vi "MagBoard_Processor.vi"() -> ()   [LabVIEW 2018]
uses:
  <vilib>/Math Plots/3D Math Plots/3D Surface/3D Surface XCtrl/3D Surface.xctl
  <vilib>/Math Plots/3D Math Plots/3D Surface/3D Surface Datatype/3D Surface Datatype.lvclass
  subVIs/calibration/FGVs/FGV States.ctl
  <vilib>/Utility/file.llb/Write Delimited Spreadsheet (DBL).vi
  <vilib>/Math Plots/3D Math Plots/3D Surface/3D Surface Datatype/Public/Plot Helper (Matrix).vi
panel:
  in  "Calibration File":string="6x0-5mm"
  in  "Save Data":bool=TRUE
  in  "Export File (CSV)":path=path "C:/Users/menprc/Documents/GitHub/MagLib/MagBoard_n64_UI/MagBoard_n64_UI_LabVIEW_Client/example_data/M064_008.csv"
  in  "dT":u32=10
  in  "Tare":bool
  out "Node XYZ List":dbl[][](array[numeric])=[[-42.056, -3144.437, -23232.0], [-518.941, -325.183, -18275.84], [1216.62, -292.139, -19514.88], [1218.122, -1916.552, -21992.96], [2617.986, -1190.335, -20444.16], [-208.027, -4484.2210000000005, -19514.88], [258.344, 873.413, -19205.12], [-4699.758, -4066.665, -21373.44], [-165.971, -412.299, -24161.28], [-1390.852, 654.872, -16107.52], [519.692, -438.584, -21063.68], [-4446.671, -1839.95, -15178.24], [-2791.467, -3060.325, -17966.079999999998], [-4864.227, -3147.441, -15178.24], [-5380.164, -1542.554, -18585.6], [-829.104, -4714.778, -20753.92], [-2151.615, 1918.805, -22302.72], [-715.703, -1658.208, -21373.44], [-5288.542, -211.782, -15797.76], [-5200.675, -1924.062, -17346.559999999998], [-6355.713, -24.783, -16727.04], [-5830.764, -1267.688, -17346.559999999998], [-6334.685, -2507.589, -17036.8], [-5066.997, 553.487, -19514.88], [3860.891, 798.313, -17346.559999999998], [2385.927, -2710.359, -17346.559999999998], [573.764, -142.69, -27878.399999999998], [2370.907, 849.381, -16107.52], [1947.343, -7.51, -17656.32], [-2110.31, -343.958, -15797.76], [1126.5, -1583.859, -20753.92], [-2659.291, -2612.729, -20753.92], [-198.264, -502.419, -22302.72], [-2278.534, 1049.898, -17346.559999999998], [3332.938, 1936.078, -17346.559999999998], [-3211.276, 720.209, -17036.8], [-1516.269, 1041.637, -18275.84], [-1339.033, 228.304, -18585.6], [-4662.959, -1410.378, -18585.6], [-4996.403, -24.783, -16417.28], [1106.974, 4200.343, -20444.16], [1601.132, 2834.274, -19824.64], [-1445.675, 4241.648, -21373.44], [-953.019, 1932.323, -16727.04], [-1794.89, 2164.382, -21063.68], [-1591.369, 1783.625, -18585.6], [-2428.734, 724.715, -16727.04], [-4816.914, -1074.681, -23541.76], [1203.102, -101.385, -23541.76], [-2397.192, 482.142, -20753.92], [-4661.457, 7558.815, -16417.28], [-6119.148, 744.241, -16727.04], [-5919.382, -162.216, -19824.64], [-3782.036, -621.077, -15797.76], [-4665.212, -1492.237, -20134.399999999998], [-3349.46, -114.903, -17346.559999999998], [-3365.982, 4614.895, -22302.72], [-3110.642, 2824.511, -19205.12], [-2347.626, 20.277, -19514.88], [-533.21, -4829.681, -27258.879999999997], [-793.056, 5227.711, -24780.8], [-5263.759, 5650.524, -21992.96], [-3424.56, 3160.208, -18895.36], [-5248.739, 1337.531, -24161.28]]
  out "Time":u32=4294745741
  in  "stop":bool
  in  "Data File":path=path "C:/Users/menprc/Documents/GitHub/MagLib/MagBoard_n64_UI/MagBoard_n64_UI_LabVIEW_Client/example_data/M064_008_up.dat"
  out "Instantaneous Data":refnum<class "3D Plot Datatype.lvclass">[](xcontrol)
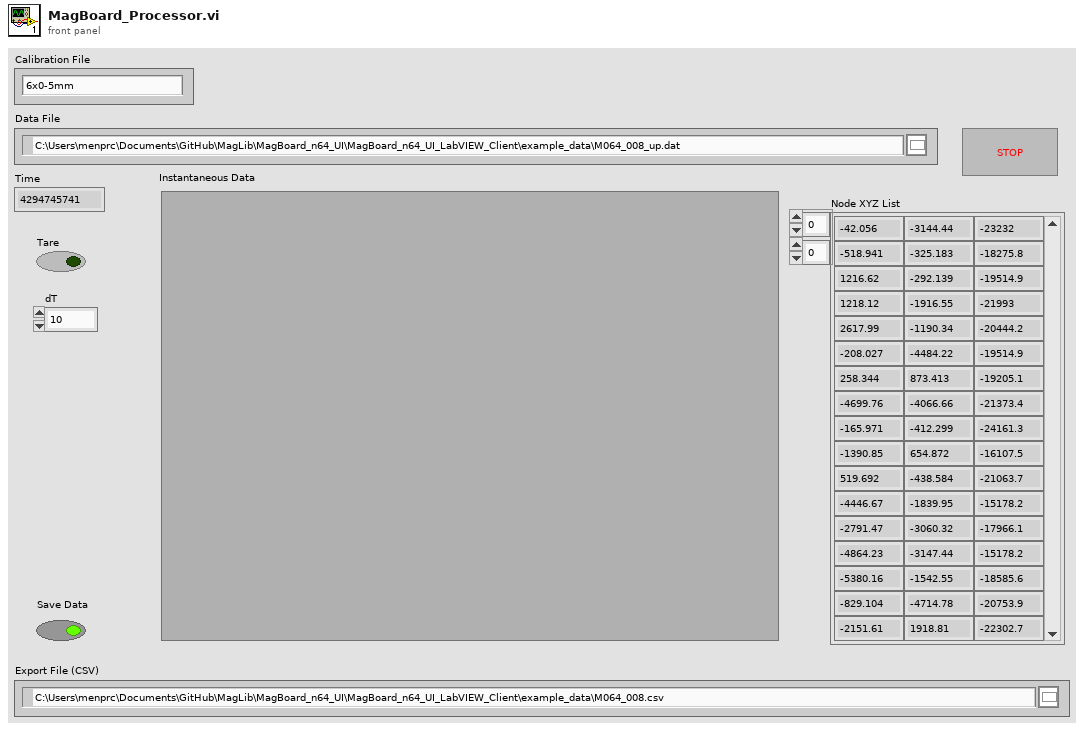
[diagram p1: front panel]
types:
  T1 = typedef "FGV States.ctl" = enum16{"Get", "Set", "Reset"}
  T2 = cluster{cluster{dbl[][], "Array":dbl[][]}, cluster{dbl[][], "Array":dbl[][]}, cluster{dbl[][], "Array":dbl[][]}, cluster{dbl[][], "Array":dbl[][]}}
  T3 = cluster{cluster{dbl[][], "Array":dbl[][]}, cluster{dbl[][], "Array":dbl[][]}, cluster{dbl[][], "Array":dbl[][]}, cluster{dbl[][], "Array":dbl[][]}}[]
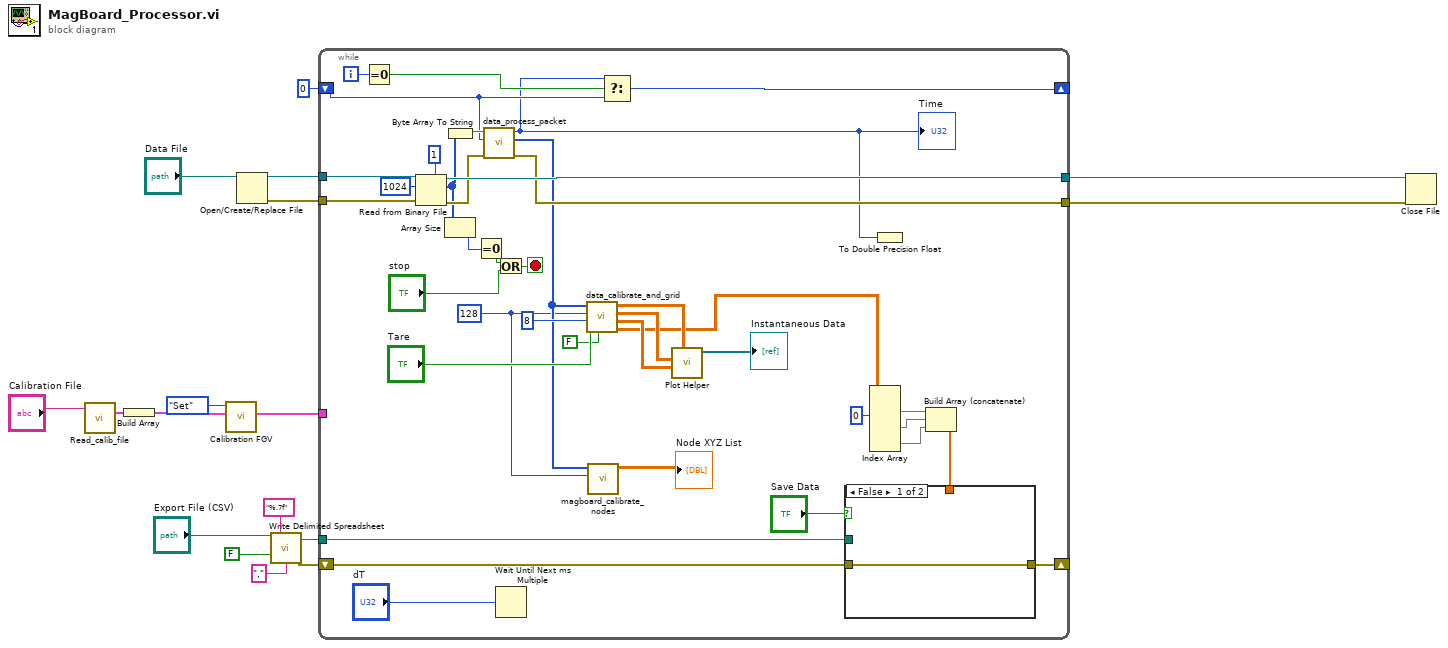
[diagram p0: block diagram]
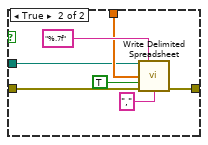
[diagram p2: hidden frame]
diagram:
  n1 = call "Read_calib_file.vi"("string"="Calibration File") -> ("output cluster"=w4:T2)  [unwired: 6 in, 4 out]
  n2 = Build Array(w4) -> (w3:T3)
  n3 = call "Calibration FGV.vi"("Calib in"=w3, "FGV States"=FGV_States."Set") -> ("Calib in 2"=w1:T3)  [unwired: 9 in]
  n4 = Open/Create/Replace File(file path (use dialog)="Data File") -> (refnum out=w16:refnum<file>, error out=w15:errorcluster)  [unwired: 5 in, 1 out]
  n5 = call-poly <vilib>:"Write Delimited Spreadsheet.vi"("file path (dialog if empty)"="Export File (CSV)", "format (%.3f)"="%.7f", "append to file? (new file:F)"=FALSE, "delimiter (\\t)"="," ("delimiter (\\t)")) -> ("new file path (Not A Path if cancelled)"=w8:path, "error out"=w6:errorcluster)  [unwired: 10 in]
  n6 = while {
    tunnel: w16 -> [w56]
    tunnel: w15 -> [w55]
    tunnel: [w53] -> w13
    tunnel: [w48] -> w14
    shift-right: [w47] -> _
    shift-left: u32 0 ("Time") -> [w45]
    tunnel: w8 -> [w30]
    shift-right: [w28] -> _
    shift-left: w6 -> [w29]
    tunnel: w1 -> [_]
    i -> [w46]
    stop <- w23 stop-if-true
    w19 = 128 ("No. Nodes")
    n7 = Equal To 0?(x=w46) -> (x = 0?=w41:bool)
    n8 = Read from Binary File(5:u8 1 ("count (1)"), 8:w55, 10:1024 ("count (1)"), 11:w56) -> (0:w49:errorcluster, 2:w26:u8[], 3:w53:refnum<file>)  [unwired: 2 in, 1 out]
    n9 = Byte Array To String(unsigned byte array=w26) -> (string=w50:string)
    n10 = Array Size(array=w26) -> (size(s)=w25:i32)
    n11 = Equal To 0?(x=w25) -> (x = 0?=w24:bool)
    n12 = call "data_process_packet.vi"("error in (no error)"=w49, "T_offset"=w45, "Data Packet"=w50) -> ("error out"=w48:errorcluster, "Sensor Readings (Signed)"=w20:i16[], "Time"=w35:u32)  [unwired: 5 in, 1 out]
    "Time" <- w35
    n13 = Or(x=w24, y="stop") -> (x .or. y?=w23:bool)
    n14 = Wait Until Next ms Multiple(millisecond multiple="dT") -> ()  [unwired: 1 out]
    n15 = call "data_calibrate_and_grid.vi"("Reset"=FALSE, "Tare"="Tare", "Row Length"=8, "No. Nodes"=w19, "Sensor Readings (PACKET)"=w20) -> ("Node XYZ List"=w21:dbl[][], "Y (GRID)"=w39:dbl[][], "X (GRID)"=w40:dbl[][], "Z (GRID)"=w42:dbl[][])  [unwired: 2 in, 1 out]
    n16 = call "magboard_calibrate_nodes.vi"("No. Nodes"=w19, "Sensor Readings (PACKET)"=w20) -> ("Sensor Output - Position (mm)"=→"Node XYZ List":dbl[][])  [unwired: 9 in]
    n17 = Select(t=w35, s=w41, f=w45) -> (s? t:f=w47:u32)
    n18 = call-poly <vilib>:"Plot Helper.vi"("z matrix"=w42, "y matrix"=w39, "x matrix"=w40) -> ("3D Plot lvclass Array out"=→"Instantaneous Data":refnum<class "3D Plot Datatype.lvclass">[])  [unwired: 3 in, 5 out]
    n19 = Index Array(array=w21, index (col) #1=0 ("disabled index (col)")) -> (element #1=w34:dbl[], element #2=w33:dbl[], element #3=w32:dbl[])  [unwired: 5 in]
    n20 = To Double Precision Float(number=w35) -> ()  [unwired: 1 out]
    n21 = Build Array (concatenate)(w34, w33, w32) -> (w31:dbl[])
    n22 = case shown="False" "Save Data" {
      tunnel: w31 -> [_ w61]
      tunnel: w30 -> [_ w60]
      tunnel: w29 -> [w57 w59]
      tunnel: [w57 w58] -> w28
      frame False {
      }
      frame True {
        n23 = call-poly <vilib>:"Write Delimited Spreadsheet.vi"("file path (dialog if empty)"=w60, "format (%.3f)"="%.7f", "1D data"=w61, "append to file? (new file:F)"=TRUE, "error in (no error)"=w59, "delimiter (\\t)"="," ("delimiter (\\t)")) -> ("error out"=w58:errorcluster)  [unwired: 8 in, 1 out]
      }
    }
  }
  n24 = Close File(refnum=w13, error in=w14) -> ()  [unwired: 2 out]
